vi "Final-Count.vi"() -> ()   [LabVIEW 2024]
panel:
  in  "Image file location":path
  out "Image":T1(plugin-control)
  in  "Datele Recoltei":T2(array[cluster])
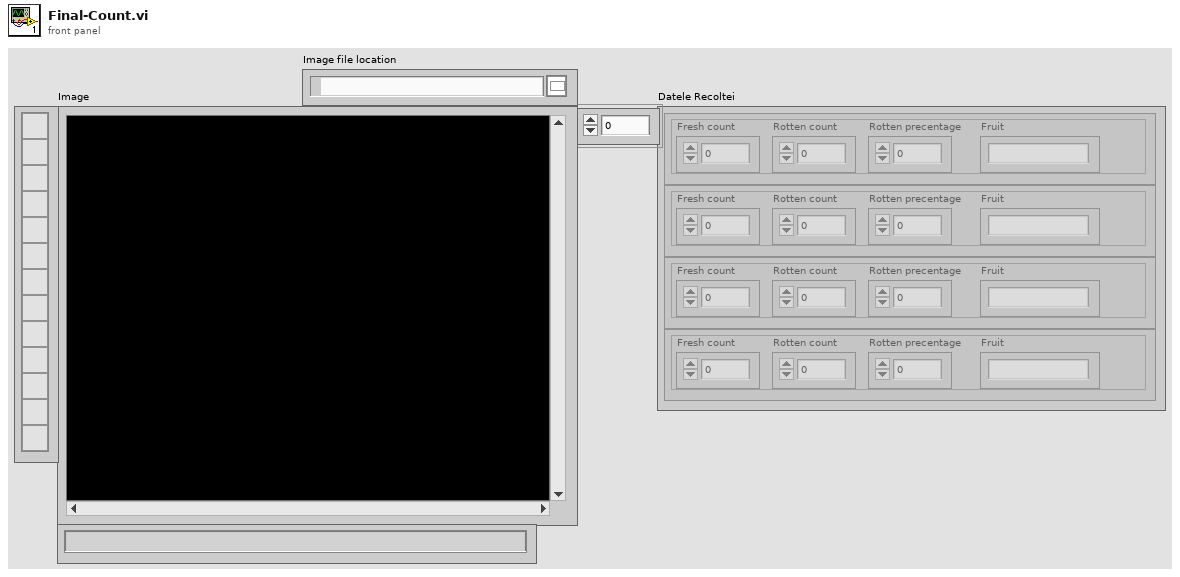
[diagram p1: front panel]
types:
  T1 = typedef "IMAQ Image.ctl" = refnum<image>
  T2 = cluster{"Fresh count":dbl, "Rotten count":dbl, "Rotten precentage":dbl, "Fruit":string}[]
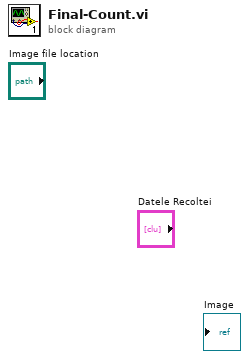
[diagram p0: block diagram]
diagram:
